vi "HighSpeedNegate.vi"(8 "input valid":bool=TRUE, 11 "x":fxp<+/-,16,14>) -> (0 "output valid":bool, 3 "-x":fxp<+/-,16,14>)   [LabVIEW 2018]
uses:
  <vilib>/rvi/FXPMathLib/FxpConvert/subVIs/nifxpmath_Convert_SimConfig.ctl
  <vilib>/fxp/LVFixedPointQuantizationPolicyTypeDef.ctl
  <vilib>/fxp/LVFixedPointOverflowPolicyTypeDef.ctl
  <vilib>/rvi/FXPMathLib/FxpConvert/simVIs/DllFxpConvertTemp_sub.vi
  <vilib>/rvi/FXPMathLib/FxpConvert/XNode/nifxpmath_Convert.xnode
  <vilib>/rvi/FXPMathLib/FxpSub/XNode/nifxpmath_Sub.xnode
  <vilib>/rvi/FXPMathLib/sim/FxpSim.dll
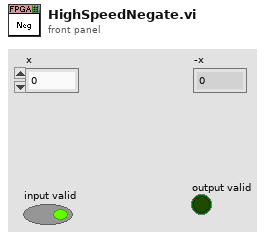
[diagram p1: front panel]
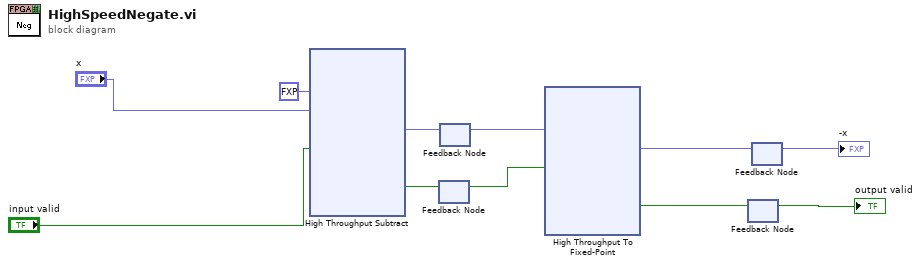
[diagram p0: block diagram]
diagram:
  n1 = xnode "High Throughput Subtract"("x"=fxp<+/-,16,14> 0.0, "y"="x", "input valid"="input valid") -> ("x-y"=w8:fxp<+/-,17,15>, "output valid"=w7:bool)  [unwired: 1 in, 1 out]
  n2 = feedback #1() -> (w11:bool)  [unwired: 1 in]
  n3 = feedback-in #1(w7) -> ()
  n4 = feedback #2() -> (w6:fxp<+/-,17,15>)  [unwired: 1 in]
  n5 = feedback-in #2(w8) -> ()
  n6 = xnode "High Throughput To Fixed-Point"("x"=w6, "input valid"=w11) -> ("y"=w5:fxp<+/-,16,14>, "output valid"=w10:bool)  [unwired: 1 in, 1 out]
  n7 = feedback #3() -> (→"output valid":bool)  [unwired: 1 in]
  n8 = feedback-in #3(w10) -> ()
  n9 = feedback #4() -> (→"-x":fxp<+/-,16,14>)  [unwired: 1 in]
  n10 = feedback-in #4(w5) -> ()
